vi "Receiver&Client.vi"() -> ()   [LabVIEW 2019]
uses:
  <instrlib>/niUSRP/niUSRP Timestamp.ctl
  <instrlib>/niUSRP/niUSRP Configure Time Start Trigger.vi
  <instrlib>/niUSRP/niUSRP Fetch Rx Data (2D CDB).vi
  <vilib>/measure/maspectr.llb/FFT Power Spectrum for 1 Chan (CDB).vi
  <vilib>/measure/NI_MAPro.lvlib
panel:
  in  "data path":path=path "D:/data/test.tdms"
  out "队列中元素数量":i32
  in  "Number of Samples \nPer Fetch":i64=40800
  in  "Timeout":dbl=10.0
  in  "Stop":bool
  out "Actual Rx Timestamp":T1
  out "IQ Graph":dbl[][](graph)
  out "Baseband Power Spectrum":cluster{"f0":dbl, "df":dbl, "magnitude":dbl[]}[](graph)
  in  "Enabled Channels":string="0,1"
  out "error out":errorcluster
  in  "Channel 1\nActive Antenna":string="RX1"
  in  "Channel 1 Gain":dbl=10.0 format="%#_6f"
  in  "Channel 0 \nActive Antenna":string="RX1"
  in  "Channel 0 Gain":dbl=10.0 format="%#_6f"
  in  "Tab Control":T2(tab)
  in  "Channel 0 Carrier\n Frequency [Hz]":dbl=2400000000.0 format="%#_6p"
  in  "Channel 1 Carrier\n Frequency [Hz]":dbl=2400000000.0 format="%#_6p"
  in  "Channel 0 Carrier\n Frequency [Hz] 2":dbl=2000000000.0 format="%#_6p"
  in  "Channel 1 Carrier\n Frequency [Hz] 2":dbl=2000000000.0 format="%#_6p"
  in  "Channel 3 Carrier\n  Frequency [Hz]":dbl=2000000000.0 format="%#_6p"
  in  "Channel 2 Carrier\n Frequency [Hz]":dbl=2000000000.0 format="%#_6p"
  in  "Carrier Frequency [Hz]":dbl=2524950000.0 format="%#_6p"
  in  "Channel 2\nActive Antenna":string="RX1"
  in  "Channel 3\nActive Antenna":string="RX1"
  in  "Channel 2 Gain":dbl=10.0 format="%#_6f"
  in  "Channel 3 Gain":dbl=10.0 format="%#_6f"
  in  "Start Trigger Time":T1={"whole seconds"=1, "fractional seconds"=0.0}
  in  "IQ Rate [S/sec]":dbl=3840000.0 format="%#_6p"
  in  "Device Name":refnum<k15>="b210mini"
  # "2974改这个配置项"
  # "b210改这个配置项"
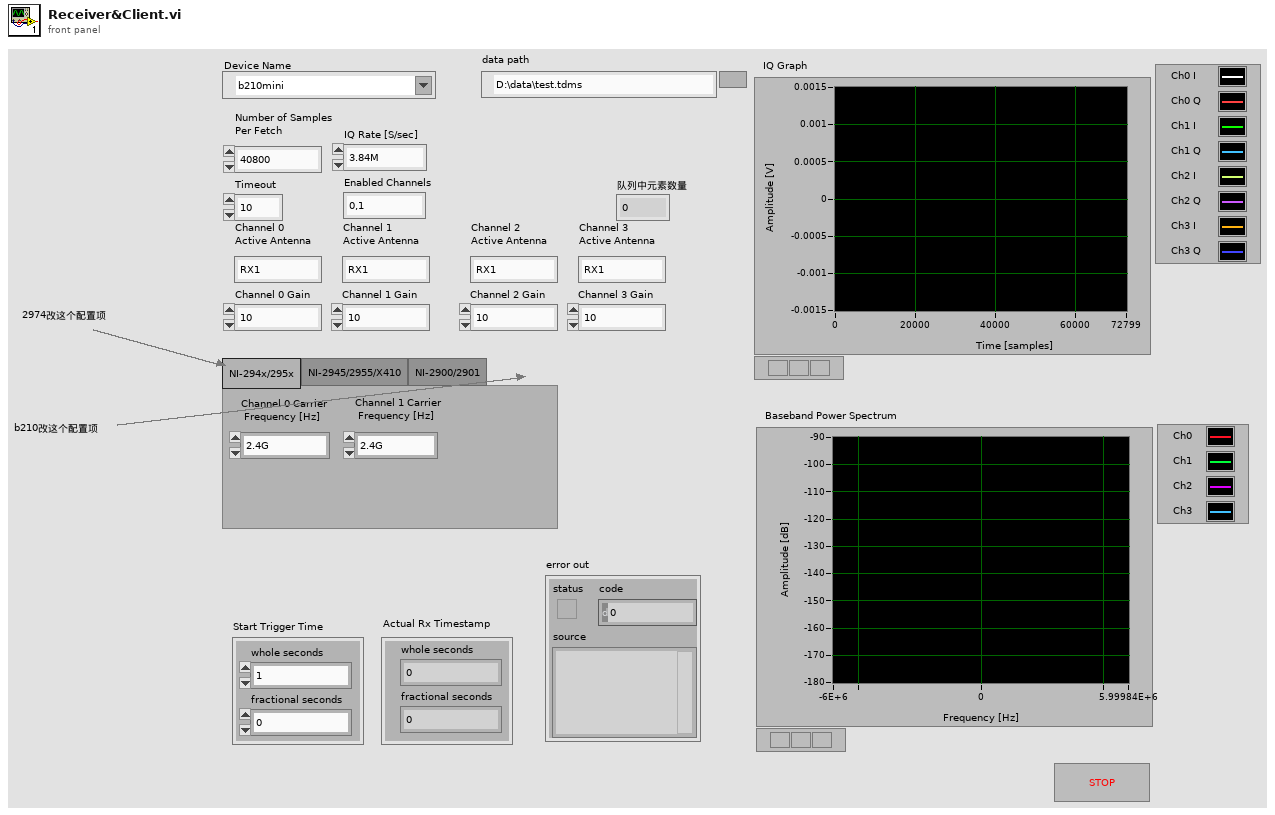
[diagram p1: front panel]
types:
  T1 = typedef "niUSRP Timestamp.ctl" = cluster{"whole seconds":u64, "fractional seconds":dbl}
  T2 = enum32{"NI-294x/295x", "NI-2945/2955/X410", "NI-2900/2901"}
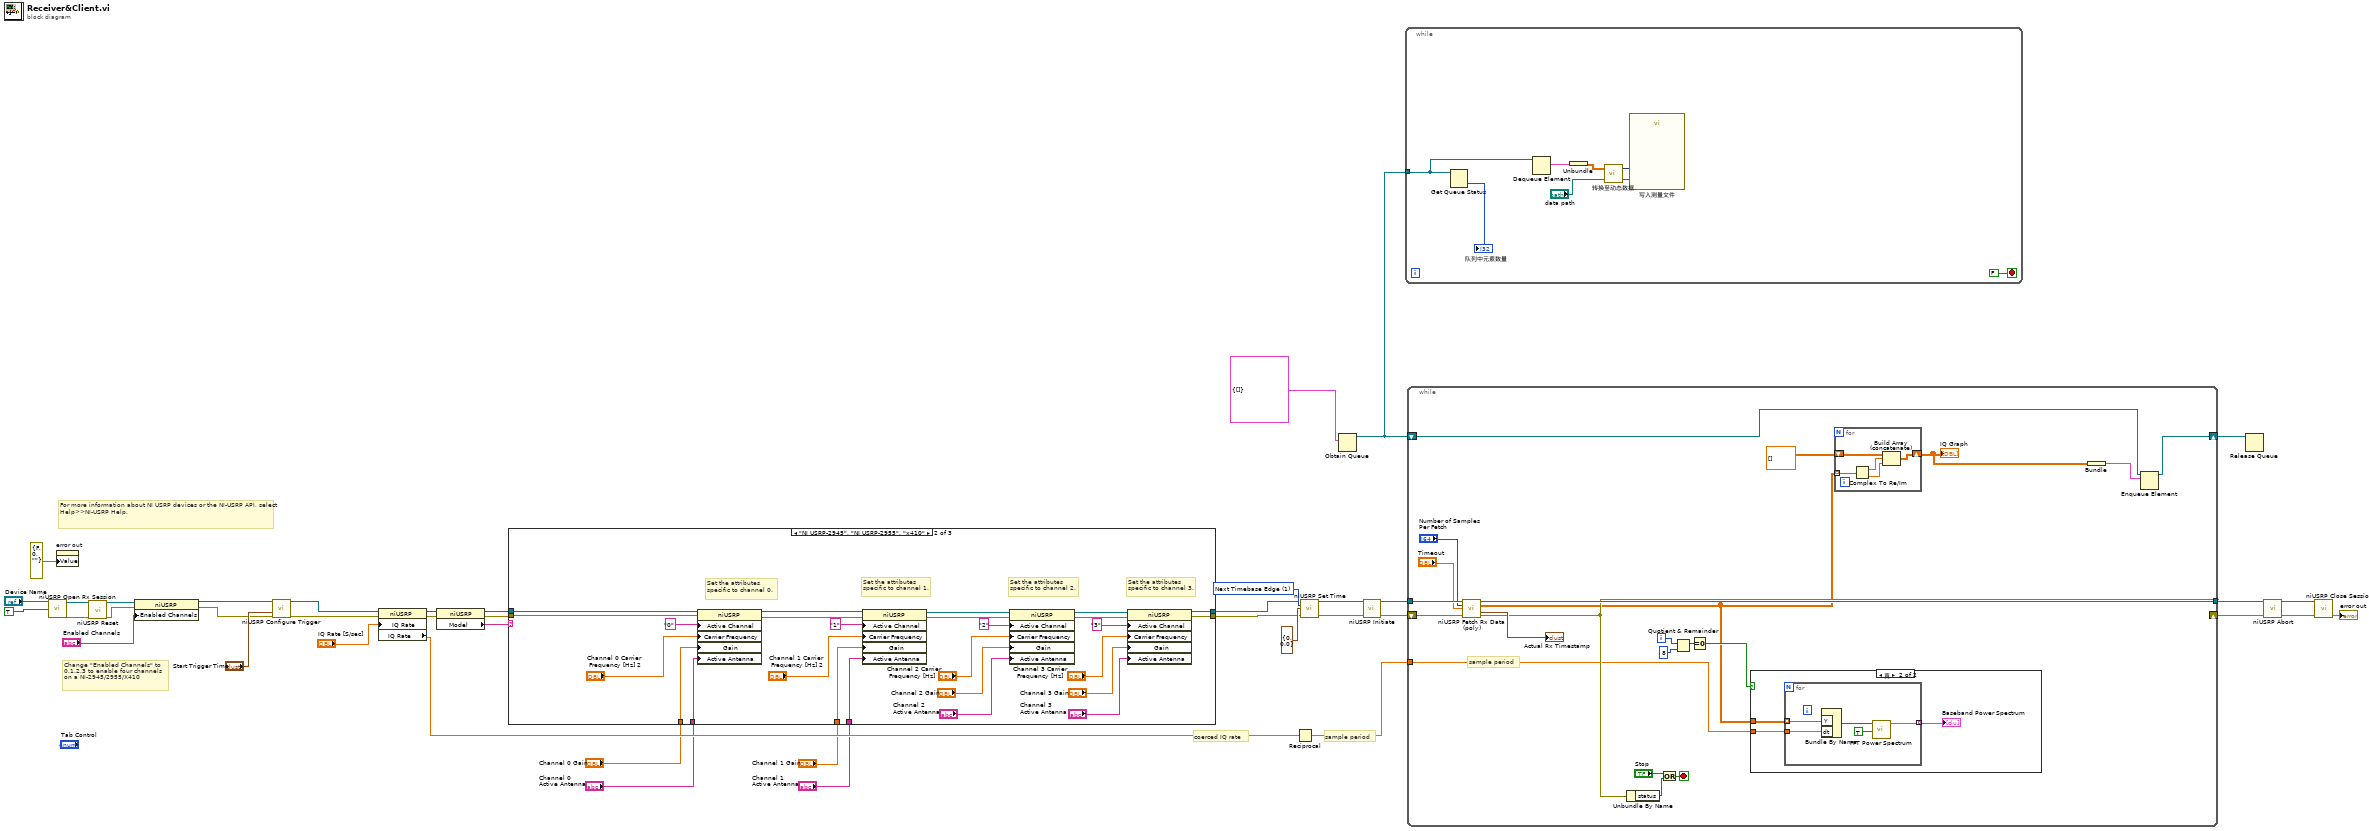
[diagram p0: block diagram]
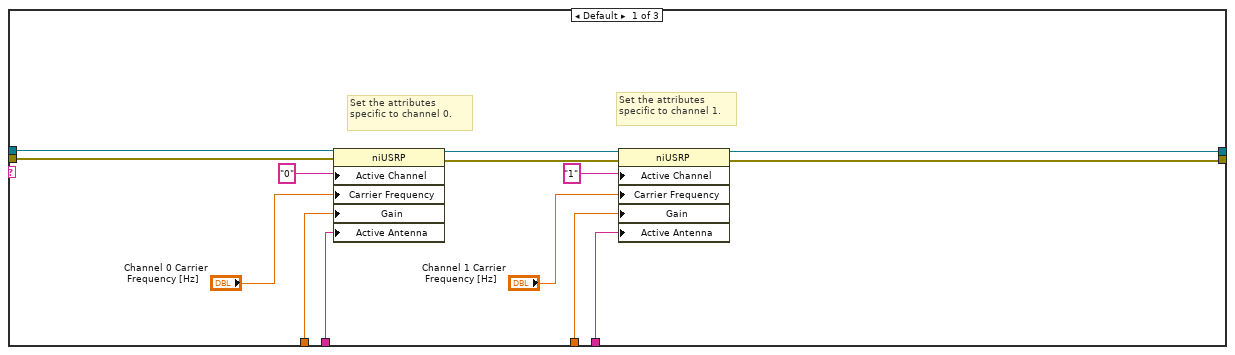
[diagram p3: hidden frame]
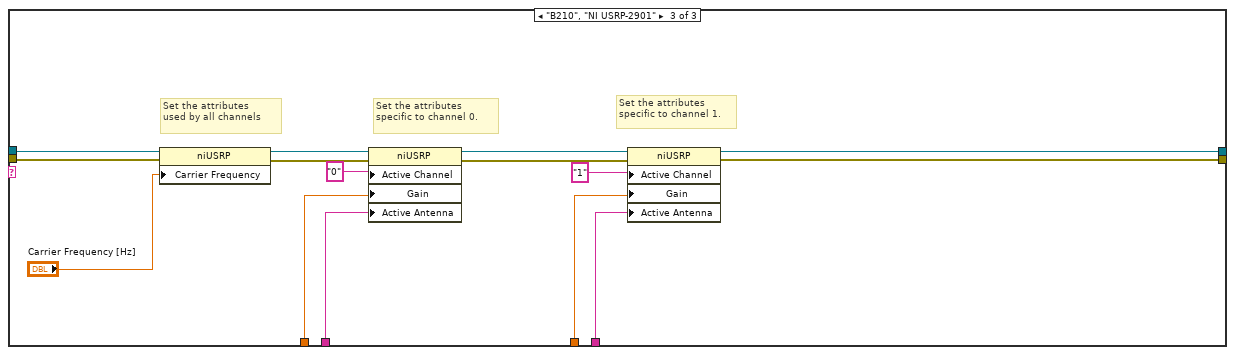
[diagram p4: hidden frame]
diagram:
  w33 = 1 items=["Now", "Next Timebase Edge"] ("apply timestamp")
  # "Change \"Enabled Channels\" to\n0,1,2,3 to enable four channels\non a NI-2945/2955/X410"
  # "For more information about NI USRP devices or the NI-USRP API, select Help>>NI-USRP Help."
  # "sample period"
  # "coerced IQ rate"
  n1 = call <instrlib>:"niUSRP Open Rx Session.vi"("device names"="Device Name", "reset"=TRUE) -> ("session handle out"=w13:refnum<k15>, "error out"=w10:errorcluster)  [unwired: 12 in]
  n2 = property on="error out" class="Clust (严格)"("Value"=errorcluster {"status"=FALSE, "code"=0, "source"=""} ("error out")) -> ()  [unwired: 2 in, 2 out]
  n3 = call <instrlib>:"niUSRP Reset.vi"("session handle"=w13, "error in (no error)"=w10) -> ("session handle out"=w12:refnum<k15>, "error out"=w11:errorcluster)  [unwired: 12 in]
  n4 = property class="niUSRP"(reference=w12, error in=w11, "Enabled Channels"="Enabled Channels") -> (reference out=w31:refnum<k15>, error out=w30:errorcluster)
  n5 = call-poly <instrlib>:"niUSRP Configure Trigger.vi"("session handle"=w31, "start trigger time"="Start Trigger Time", "error in (no error)"=w30) -> ("session handle out"=w29:refnum<k15>, "error out"=w28:errorcluster)  [unwired: 11 in]
  n6 = property class="niUSRP"(reference=w29, error in=w28, "IQ Rate"="IQ Rate [S/sec]") -> (reference out=w24:refnum<k15>, error out=w26:errorcluster, "IQ Rate"=w39:dbl)
  n7 = property class="niUSRP"(reference=w24, error in=w26) -> (reference out=w23:refnum<k15>, error out=w25:errorcluster, "Model"=w27:string)
  n8 = case shown="\"NI USRP-2945\", \"NI USRP-2955\", \"x410\"" w27 {
    tunnel: w25 -> [w51 w77 w86]
    tunnel: w23 -> [w50 w76 w87]
    tunnel: [w49 w69 w92] -> w18
    tunnel: [w48 w68 w82] -> w17
    tunnel: "Channel 0 Gain" -> [w47 w75 w91]
    tunnel: "Channel 0 \nActive Antenna" -> [w46 w74 w90]
    tunnel: "Channel 1 Gain" -> [w45 w73 w89]
    tunnel: "Channel 1\nActive Antenna" -> [w44 w72 w88]
    frame Default {
      # "Set the attributes \nspecific to channel 1."
      # "Set the attributes \nspecific to channel 0."
      n9 = property class="niUSRP"(reference=w50, error in=w51, "Active Channel"="0", "Carrier Frequency"="Channel 0 Carrier\n Frequency [Hz]", "Gain"=w47, "Active Antenna"=w46) -> (reference out=w55:refnum<k15>, error out=w54:errorcluster)
      n10 = property class="niUSRP"(reference=w55, error in=w54, "Active Channel"="1", "Carrier Frequency"="Channel 1 Carrier\n Frequency [Hz]", "Gain"=w45, "Active Antenna"=w44) -> (reference out=w49:refnum<k15>, error out=w48:errorcluster)
    }
    frame "NI USRP-2945", "NI USRP-2955", "x410" {
      # "Set the attributes \nspecific to channel 3."
      # "Set the attributes \nspecific to channel 2."
      # "Set the attributes \nspecific to channel 1."
      # "Set the attributes \nspecific to channel 0."
      n11 = property class="niUSRP"(reference=w76, error in=w77, "Active Channel"="0", "Carrier Frequency"="Channel 0 Carrier\n Frequency [Hz] 2", "Gain"=w75, "Active Antenna"=w74) -> (reference out=w81:refnum<k15>, error out=w80:errorcluster)
      n12 = property class="niUSRP"(reference=w81, error in=w80, "Active Channel"="1", "Carrier Frequency"="Channel 1 Carrier\n Frequency [Hz] 2", "Gain"=w73, "Active Antenna"=w72) -> (reference out=w71:refnum<k15>, error out=w66:errorcluster)
      n13 = property class="niUSRP"(reference=w71, error in=w66, "Active Channel"="2", "Carrier Frequency"="Channel 2 Carrier\n Frequency [Hz]", "Gain"="Channel 2 Gain", "Active Antenna"="Channel 2\nActive Antenna") -> (reference out=w70:refnum<k15>, error out=w67:errorcluster)
      n14 = property class="niUSRP"(reference=w70, error in=w67, "Active Channel"="3", "Carrier Frequency"="Channel 3 Carrier\n  Frequency [Hz]", "Gain"="Channel 3 Gain", "Active Antenna"="Channel 3\nActive Antenna") -> (reference out=w69:refnum<k15>, error out=w68:errorcluster)
    }
    frame "B210", "NI USRP-2901" {
      # "Set the attributes \nused by all channels"
      # "Set the attributes \nspecific to channel 1."
      # "Set the attributes \nspecific to channel 0."
      n15 = property class="niUSRP"(reference=w87, error in=w86, "Carrier Frequency"="Carrier Frequency [Hz]") -> (reference out=w85:refnum<k15>, error out=w84:errorcluster)
      n16 = property class="niUSRP"(reference=w85, error in=w84, "Active Channel"="0", "Gain"=w91, "Active Antenna"=w90) -> (reference out=w96:refnum<k15>, error out=w95:errorcluster)
      n17 = property class="niUSRP"(reference=w96, error in=w95, "Active Channel"="1", "Gain"=w89, "Active Antenna"=w88) -> (reference out=w92:refnum<k15>, error out=w82:errorcluster)
    }
  }
  n18 = Reciprocal(x=w39) -> (1/x=w14:dbl)
  n19 = call <instrlib>:"niUSRP Set Time.vi"("session handle"=w18, "apply timestamp"=w33, "timestamp"=T1 {"whole seconds"=0, "fractional seconds"=0.0}, "error in (no error)"=w17) -> ("session handle out"=w35:refnum<k15>, "error out"=w34:errorcluster)  [unwired: 10 in]
  n20 = Obtain Queue(element data type=cluster{dbl[][]} {[]}) -> (queue out=w6:refnum<queue>)  [unwired: 4 in, 2 out]
  n21 = call <instrlib>:"niUSRP Initiate.vi"("session handle"=w35, "error in (no error)"=w34) -> ("session handle out"=w15:refnum<k15>, "error out"=w16:errorcluster)  [unwired: 12 in]
  n22 = while {
    tunnel: w6 -> [w103]
    stop <- FALSE stop-if-true
    n23 = Get Queue Status(queue=w103) -> (# elements in queue=→"队列中元素数量":i32)  [unwired: 2 in, 7 out]
    n24 = Dequeue Element(queue=w103) -> (element=w101:cluster{dbl[][]})  [unwired: 2 in, 3 out]
    n25 = Unbundle(w101) -> (w100:dbl[][])
    n26 = call "转换至动态数据"("2D Array"=w100) -> ("Dynamic Data Type"=w99:dynamicdata)  [unwired: 3 in]
    n27 = call "写入测量文件"("Signals"=w99, "Filename"="data path") -> ()  [unwired: 15 in, 3 out]
  }
  n28 = while {
    tunnel: w15 -> [w124]
    tunnel: [w120] -> w1
    shift-right: [w115] -> w2
    shift-left: w16 -> [w123]
    tunnel: w14 -> [w105]
    shift-right: [w113] -> w7
    shift-left: w6 -> [w114]
    i -> [w108]
    stop <- w119 stop-if-true
    # "sample period"
    n29 = call-poly <instrlib>:"niUSRP Fetch Rx Data (poly).vi"("session handle"=w124, "number of samples"="Number of Samples \nPer Fetch", "timeout"="Timeout", "error in (no error)"=w123) -> ("session handle out"=w120:refnum<k15>, "data"=w106:cdb[][], "timestamp"=→"Actual Rx Timestamp":T1, "error out"=w115:errorcluster)  [unwired: 8 in]
    n30 = Unbundle By Name(w115) -> ("status"=w117:bool)
    n31 = Or(x="Stop", y=w117) -> (x .or. y?=w119:bool)
    n32 = Quotient & Remainder(x=w108, y=8) -> (x-y*floor(x/y)=w110:i32)  [unwired: 1 out]
    n33 = Equal To 0?(x=w110) -> (x = 0?=w107:bool)
    n34 = case shown="真" w107 {
      tunnel: w106 -> [_ w127]
      tunnel: w105 -> [_ w126]
      frame False {
      }
      frame True {
        n35 = for {
          tunnel: [w132] -> w125 mode=indexing
          tunnel: w127 -> [w130] mode=indexing
          tunnel: w126 -> [w128]
          n36 = Bundle By Name("Y"=w130, "dt"=w128) -> (w129:waveform(cdb))  [unwired: 1 in]
          n37 = call-poly <vilib>:"FFT Power Spectrum.vi"("dB On (F)"=TRUE, "time signal"=w129) -> ("power spectrum"=w132:cluster{"f0":dbl, "df":dbl, "magnitude":dbl[]})  [unwired: 6 in, 3 out]
        }
        "Baseband Power Spectrum" <- w125
      }
    }
    n38 = for {
      tunnel: w106 -> [w137] mode=indexing
      shift-right: [w134] -> w111
      shift-left: dbl[][] [] -> [w133]
      n39 = Complex To Re/Im(x + iy=w137) -> (x=w136:dbl[], y=w135:dbl[])
      n40 = Build Array (concatenate)(w133, w136, w135) -> (w134:dbl[][])
    }
    "IQ Graph" <- w111
    n41 = Bundle(w111) -> (w104:cluster{dbl[][]})  [unwired: 1 in]
    n42 = Enqueue Element(queue=w114, element=w104) -> (queue out=w113:refnum<queue>)  [unwired: 2 in, 2 out]
  }
  n43 = Release Queue(queue=w7) -> ()  [unwired: 2 in, 3 out]
  n44 = call <instrlib>:"niUSRP Abort.vi"("session handle"=w1, "error in (no error)"=w2) -> ("session handle out"=w4:refnum<k15>, "error out"=w5:errorcluster)  [unwired: 12 in]
  n45 = call <instrlib>:"niUSRP Close Session.vi"("session handle"=w4, "error in (no error)"=w5) -> ("error out"=→"error out":errorcluster)  [unwired: 13 in]
